vi "shm info init.vi"(8 "error in (no error)":errorcluster, 10 "shared memory configuration in":refnum<class "Shared Memory configuration.lvclass">, 11 "shared memory runtime in":refnum<class "Shared Memory runtime.lvclass">) -> (0 "error out":errorcluster, 2 "shared memory configuration out":refnum<class "Shared Memory configuration.lvclass">, 3 "shared memory runtime out":refnum<class "Shared Memory runtime.lvclass">)   [LabVIEW 2013, in "Shared Memory runtime.lvclass"]
uses:
  Shared Memory runtime.lvclass
  configuration/Shared Memory configuration.lvclass
  controls/shm info.ctl
  <vilib>/NI/Shared Memory Library/Classes/Shared Memory/Public/Controls/reference.ctl
  <vilib>/NI/Shared Memory Library/Classes/Shared Memory/Shared Memory.lvclass
  controls/shm info ptrs.ctl
  configuration/Shared Memory configuration.lvclass/Shared Memory configuration.ctl
  <vilib>/NI/Shared Memory Library/Classes/Shared Memory/Public/Controls/permissions group.ctl
  <vilib>/NI/Shared Memory Library/Classes/Shared Memory/Public/Controls/permissions.ctl
  Shared Memory runtime.lvclass/Shared Memory runtime.ctl
  <vilib>/NI/Shared Memory Library/Pointer Operations/Write Scalar U8.vi
  configuration/Read engine info shm name.vi
  configuration/Read revision major.vi
  configuration/Read header minor.vi
  Write shm info.vi
  <vilib>/NI/Shared Memory Library/Shared Memory.lvlib
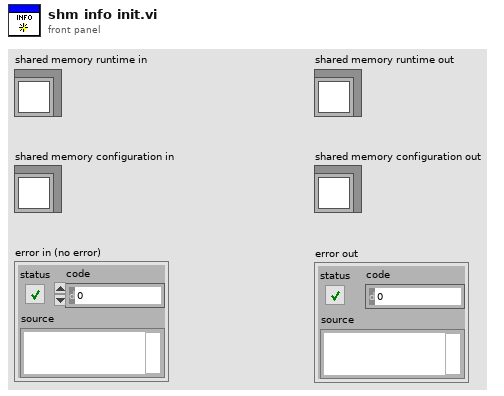
[diagram p1: front panel]
types:
  T1 = typedef "Shared Memory runtime.lvclass/shm info.ctl" = cluster{"shared memory":T2, "shm info ptrs":T3, "created?":bool}
  T2 = typedef "Shared Memory.lvlib/Shared Memory.lvclass/reference.ctl" = refnum<data-value>
  T3 = typedef "Shared Memory runtime.lvclass/shm info ptrs.ctl" = cluster{"rev_major_ptr":u64, "rev_minor_ptr":u64}
  T4 = typedef "Shared Memory.lvlib/Shared Memory.lvclass/permissions group.ctl" = cluster{"owner":T5, "group":T5, "everyone":T5}
  T5 = typedef "Shared Memory.lvlib/Shared Memory.lvclass/permissions.ctl" = cluster{"read":bool, "write":bool, "execute":bool}
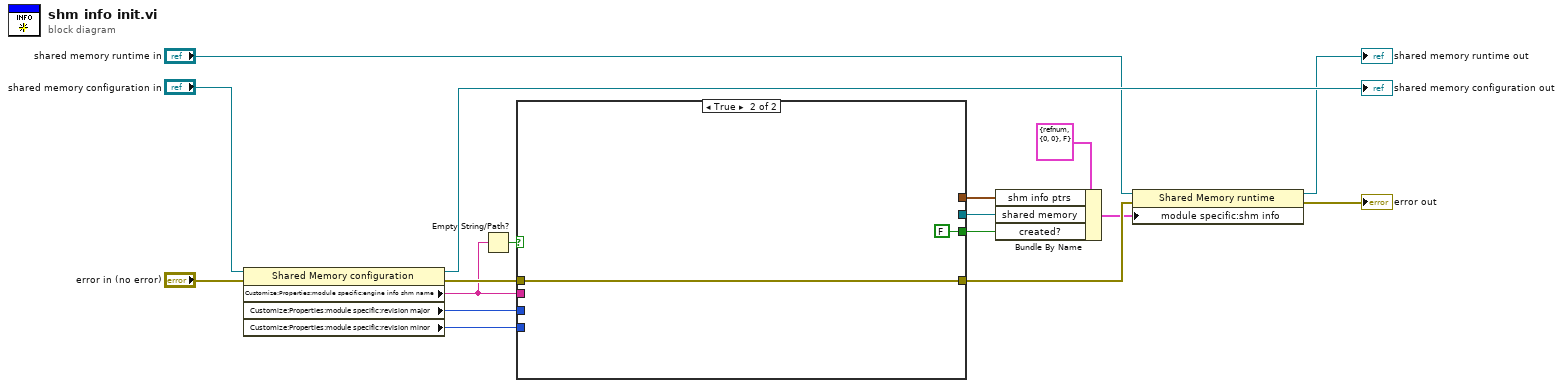
[diagram p0: block diagram]
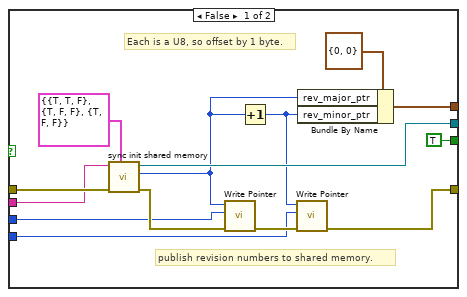
[diagram p2: hidden frame]
diagram:
  n1 = property class="Shared Memory configuration"(reference="shared memory configuration in", error in="error in (no error)") -> (reference out=→"shared memory configuration out":refnum<class "Shared Memory configuration.lvclass">, error out=w11:errorcluster, "Customize:Properties:module specific:engine info shm name"=w3:string, "Customize:Properties:module specific:revision major"=w7:u8, "Customize:Properties:module specific:revision minor"=w4:u8)
  n2 = Empty String/Path?(string/path=w3) -> (empty?=w2:bool)
  n3 = case shown="True" w2 {
    tunnel: w11 -> [w31 w33]
    tunnel: w3 -> [w30 _]
    tunnel: [w27 _] -> w9
    tunnel: [w26 _] -> w8
    tunnel: w7 -> [w23 _]
    tunnel: [w20 w33] -> w6
    tunnel: w4 -> [w19 _]
    tunnel: [TRUE FALSE] -> w1
    frame False {
      # "publish revision numbers to shared memory."
      # "Each is a U8, so offset by 1 byte."
      n4 = call "sync init shared memory.vi"("permissions (0664)"=T4 {"owner"={"read"=TRUE, "write"=TRUE, "execute"=FALSE}, "group"={"read"=TRUE, "write"=FALSE, "execute"=FALSE}, "everyone"={"read"=TRUE, "write"=FALSE, "execute"=FALSE}}, "error in (no error)"=w31, "sync shm name"=w30) -> ("error out"=w25:errorcluster, "pointer to shared memory"=w24:u64, "shared memory out"=w27:T2)  [unwired: 6 in]
      n5 = call-poly <vilib>:"Write Pointer.vi"("error in (no error)"=w25, "value"=w23, "pointer in"=w24) -> ("error out"=w22:errorcluster)  [unwired: 7 in, 1 out]
      n6 = Increment(x=w24) -> (x+1=w21:u64)
      n7 = call-poly <vilib>:"Write Pointer.vi"("error in (no error)"=w22, "value"=w19, "pointer in"=w21) -> ("error out"=w20:errorcluster)  [unwired: 7 in, 1 out]
      n8 = Bundle By Name(cluster=T3 {"rev_major_ptr"=0, "rev_minor_ptr"=0} ("shm info ptrs"), "rev_major_ptr"=w24, "rev_minor_ptr"=w21) -> (w26:T3)
    }
    frame True {
    }
  }
  n9 = Bundle By Name(cluster=T1 {"shared memory"=refnum, "shm info ptrs"={"rev_major_ptr"=0, "rev_minor_ptr"=0}, "created?"=FALSE} ("shm info"), "shm info ptrs"=w8, "shared memory"=w9, "created?"=w1) -> (w5:T1)
  n10 = property class="Shared Memory runtime"(reference="shared memory runtime in", error in=w6, "module specific:shm info"=w5) -> (reference out=→"shared memory runtime out":refnum<class "Shared Memory runtime.lvclass">, error out=→"error out":errorcluster)
